vi "Untitled 5.vi"() -> ()   [LabVIEW 2017]
uses:
  Global 1.vi
panel:
  in  "Boolean":bool
  out "Numeric":i32
  out "지호씨가보낸 총좌표":string
  in  "stop":bool
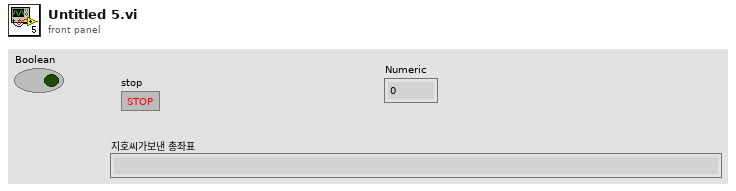
[diagram p1: front panel]
types:
  T1 = enum16{"Standard", "Buffered", "CRLF", "Immediate"}
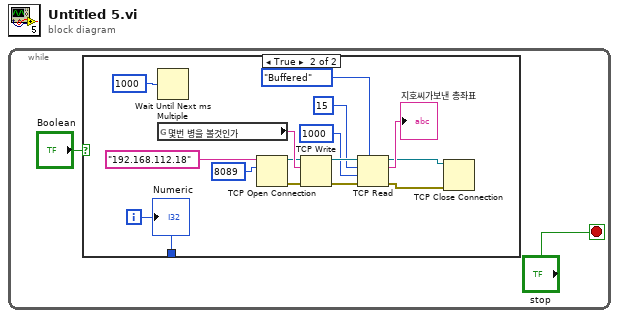
[diagram p0: block diagram]
diagram:
  n1 = while {
    i -> [w2]
    stop <- "stop" stop-if-true
    n2 = case shown="True" "Boolean" {
      tunnel: w2 -> [_ w10]
      frame False {
      }
      frame True {
        n3 = Wait Until Next ms Multiple(millisecond multiple=u32 1000 ("milliseconds to wait")) -> ()  [unwired: 1 out]
        n4 = global read "Global 1.vi" "몇번 병을 볼것인가"() -> (w16:string)
        n5 = TCP Open Connection(address="192.168.112.18", remote port or service name=u16 8089) -> (connection ID=w6:refnum<k5>, error out=w7:errorcluster)  [unwired: 3 in]
        n6 = TCP Write(connection ID=w6, data in=w16, error in (no error)=w7) -> (connection ID out=w18:refnum<k5>, error out=w17:errorcluster)  [unwired: 1 in, 1 out]
        n7 = TCP Read(connection ID=w18, bytes to read=15, error in (no error)=w17, 7:T1."Buffered" ("mode (standard)"), 9:1000 ("timeout ms (25000)")) -> (connection ID out=w4:refnum<k5>, data out=→"지호씨가보낸 총좌표":string, error out=w5:errorcluster)
        n8 = TCP Close Connection(connection ID=w4, error in (no error)=w5) -> ()  [unwired: 1 in, 2 out]
        "Numeric" <- w10
      }
    }
  }
